vi "Error 5009 - Error Opening COM Port.vi"() -> (0 "error out":errorcluster)   [LabVIEW 2021]
doc: "Error 5004 - TCP Timeout"
uses:
  <vilib>/Utility/error.llb/Error Cluster From Error Code.vi
  <vilib>/ErrorRing/Error Ring.xnode
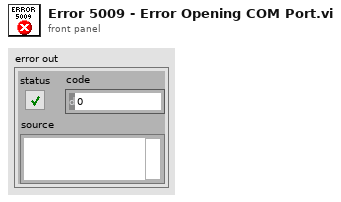
[diagram p1: front panel]
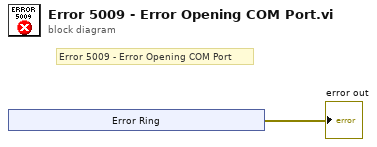
[diagram p0: block diagram]
diagram:
  # "Error 5009 - Error Opening COM Port"
  n1 = xnode "Error Ring"() -> ("error out"=→"error out":errorcluster)
